vi "2048-1.vi"() -> ()   [LabVIEW 2018]
panel:
  out "Ring 25":u16(ring)
  out "Ring 24":u16(ring)
  out "Ring 23":u16(ring)
  out "Ring 22":u16(ring)
  out "Ring 21":u16(ring)
  out "Ring 20":u16(ring)
  out "Ring 19":u16(ring)
  out "Ring 18":u16(ring)
  out "Ring 17":u16(ring)
  out "Ring 16":u16(ring)
  out "Ring 15":u16(ring)
  out "Ring 14":u16(ring)
  out "Ring 13":u16(ring)
  out "Ring 12":u16(ring)
  out "Ring 11":u16(ring)
  out "Ring 10":u16(ring)
  out "Ring 9":u16(ring)
  out "Ring 8":u16(ring)
  out "Ring 7":u16(ring)
  out "Ring 6":u16(ring)
  out "Ring 5":u16(ring)
  out "Ring 4":u16(ring)
  out "Ring 3":u16(ring)
  out "Ring 2":u16(ring)
  out "mode":i32
  in  "Type":enum16{"經典", "角落動物", "星座", "寶可夢", "彩色"}(ring)
  out "ringArray":refnum<vi>[][](array[refnum])
  out "Ring":u16(ring)
  in  "Game Over":string="Game Over"
  in  "Winner":string="Winner"
  in  "New Game":bool
  out "Score":dbl
  in  "Exit":bool
  in  "Down":bool
  in  "Up":bool
  in  "Right":bool
  in  "Left":bool
  in  "Board":i32[][](array[numeric])=[[0, 0, 0, 0], [0, 0, 0, 0], [0, 0, 0, 0], [0, 0, 0, 0]]
  in  "Ring 26":u16(ring)
  # "Overview: This example is a LabVIEW version of the number game 2048.\nRequirements: LabVIEW 2012 (or compatible)\nInstructions:\n1.Run the VI\n2.Use the the left, right, up, and down arrows to slide number"
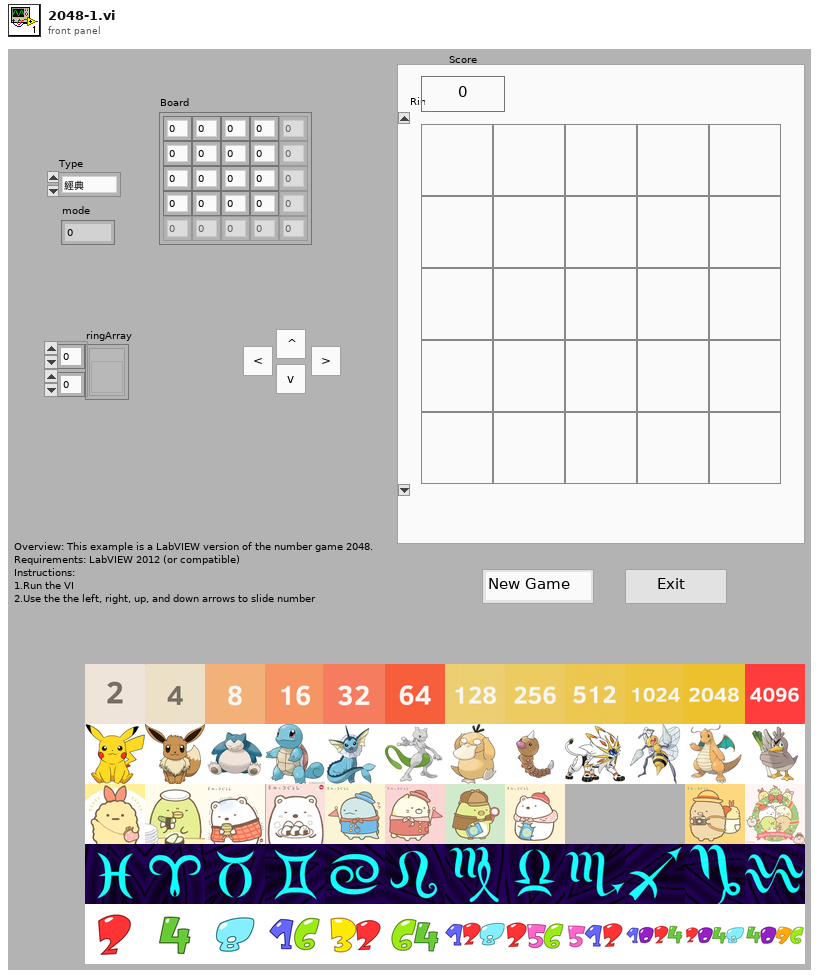
[diagram p1: front panel]
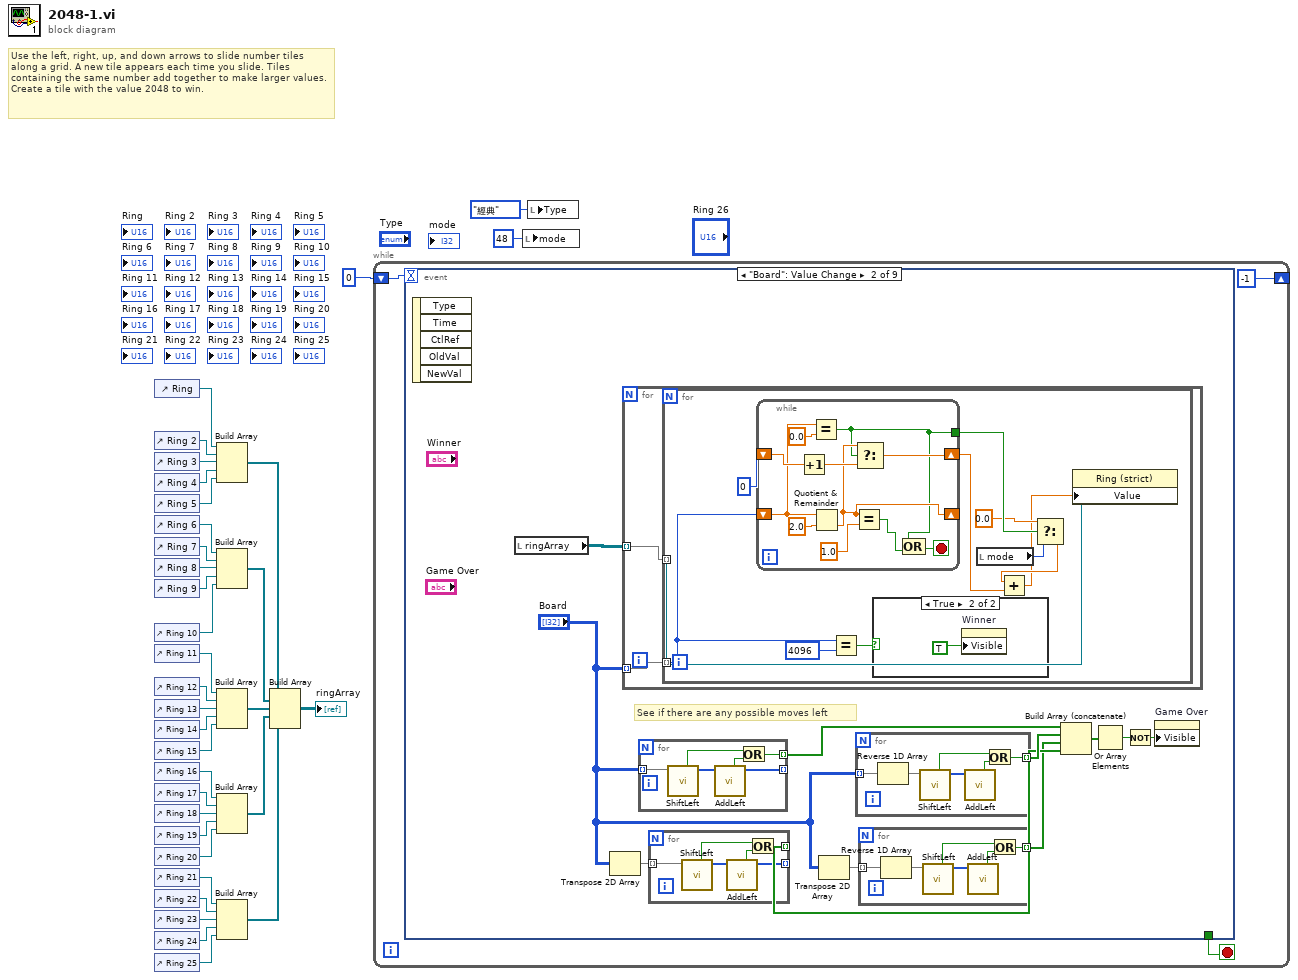
[diagram p0: block diagram]
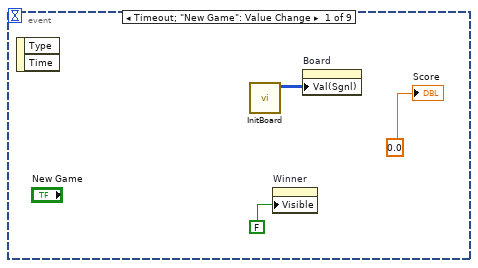
[diagram p2: hidden frame]
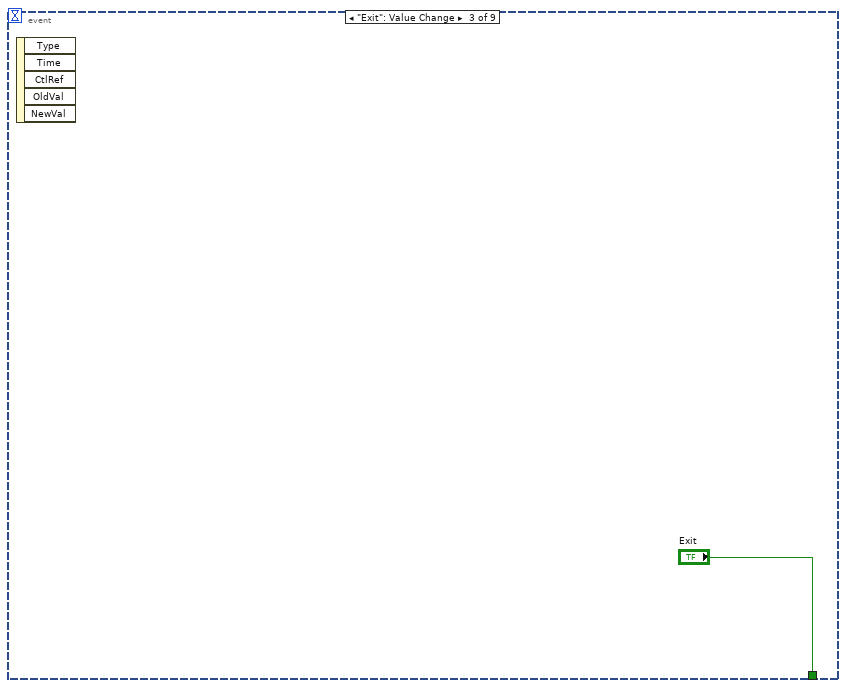
[diagram p4: hidden frame]
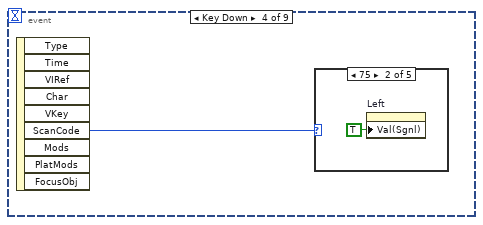
[diagram p5: hidden frame]
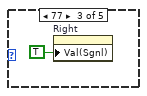
[diagram p7: hidden frame]
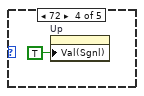
[diagram p8: hidden frame]
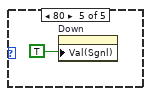
[diagram p9: hidden frame]
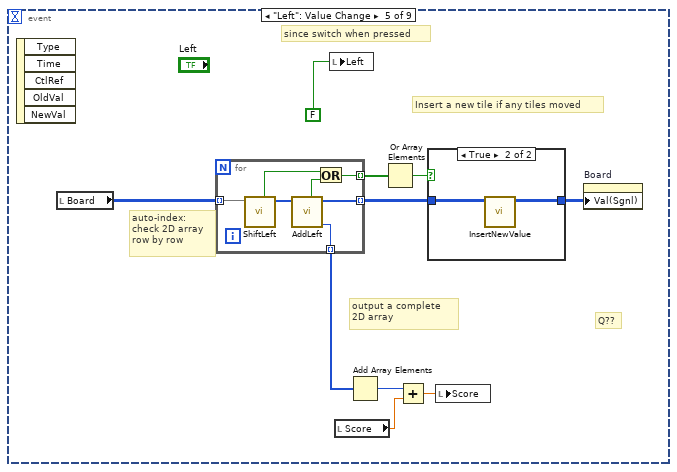
[diagram p10: hidden frame]
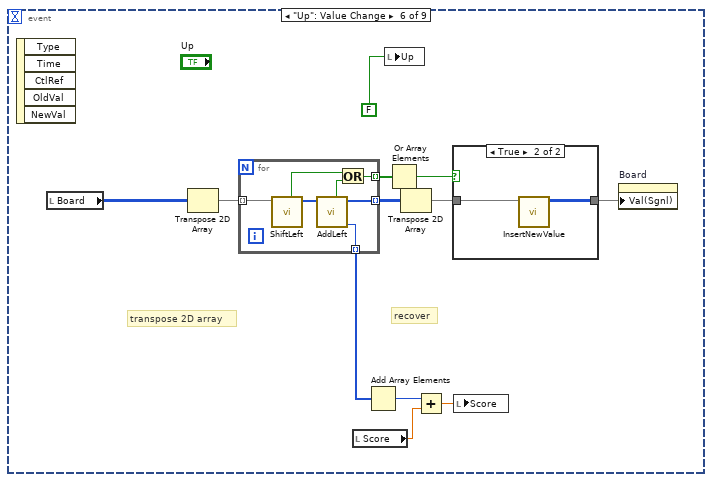
[diagram p12: hidden frame]
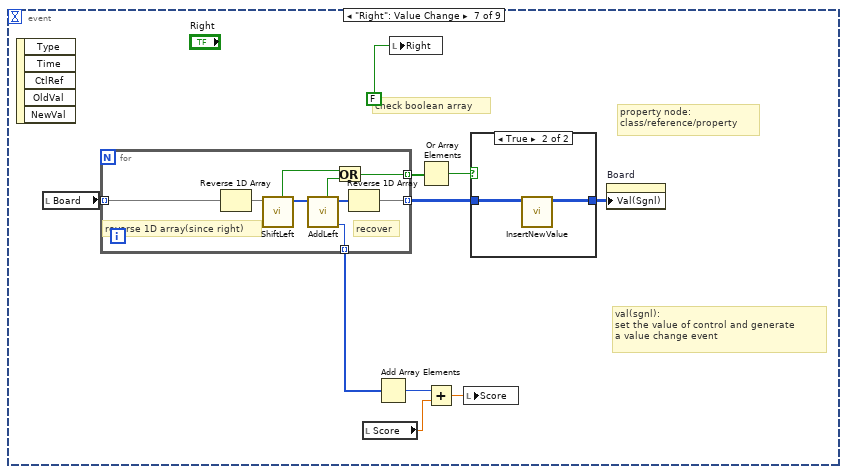
[diagram p14: hidden frame]
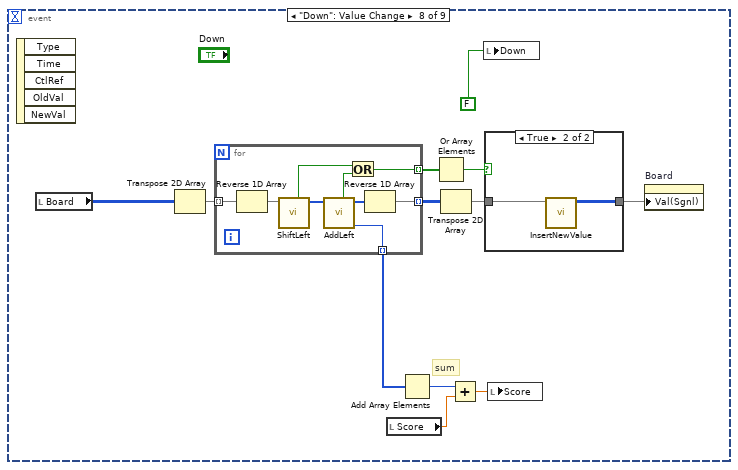
[diagram p16: hidden frame]
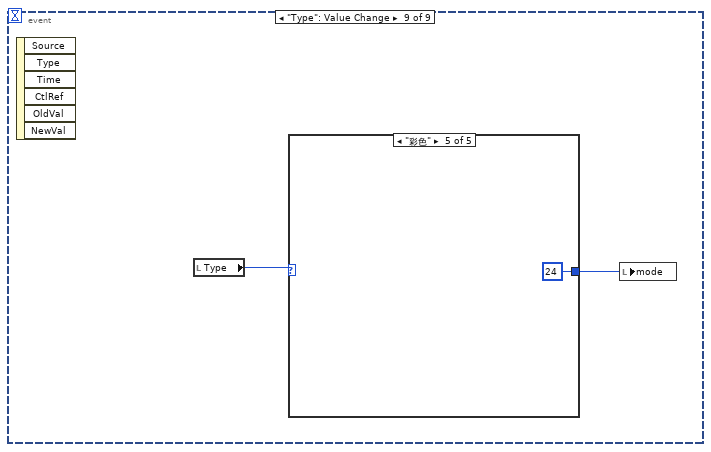
[diagram p18: hidden frame]
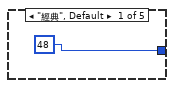
[diagram p19: hidden frame]
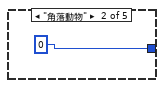
[diagram p20: hidden frame]
diagram:
  # "Use the left, right, up, and down arrows to slide number tiles along a grid. A new tile appears each time you slide. Tiles containing the same number add together to make larger values. Create a tile with the value 2048 to win."
  n1 = control-ref of="Ring"() -> (w32:refnum<vi>)
  n2 = control-ref of="Ring 2"() -> (w28:refnum<vi>)
  n3 = control-ref of="Ring 3"() -> (w29:refnum<vi>)
  n4 = control-ref of="Ring 4"() -> (w27:refnum<vi>)
  n5 = control-ref of="Ring 5"() -> (w26:refnum<vi>)
  n6 = control-ref of="Ring 6"() -> (w24:refnum<vi>)
  n7 = control-ref of="Ring 7"() -> (w23:refnum<vi>)
  n8 = control-ref of="Ring 8"() -> (w25:refnum<vi>)
  n9 = control-ref of="Ring 9"() -> (w22:refnum<vi>)
  n10 = control-ref of="Ring 10"() -> (w21:refnum<vi>)
  n11 = control-ref of="Ring 11"() -> (w20:refnum<vi>)
  n12 = control-ref of="Ring 12"() -> (w19:refnum<vi>)
  n13 = control-ref of="Ring 13"() -> (w18:refnum<vi>)
  n14 = control-ref of="Ring 14"() -> (w17:refnum<vi>)
  n15 = control-ref of="Ring 15"() -> (w16:refnum<vi>)
  n16 = control-ref of="Ring 16"() -> (w15:refnum<vi>)
  n17 = control-ref of="Ring 17"() -> (w14:refnum<vi>)
  n18 = control-ref of="Ring 18"() -> (w13:refnum<vi>)
  n19 = control-ref of="Ring 19"() -> (w12:refnum<vi>)
  n20 = control-ref of="Ring 20"() -> (w11:refnum<vi>)
  n21 = control-ref of="Ring 21"() -> (w10:refnum<vi>)
  n22 = control-ref of="Ring 22"() -> (w9:refnum<vi>)
  n23 = control-ref of="Ring 23"() -> (w8:refnum<vi>)
  n24 = control-ref of="Ring 24"() -> (w7:refnum<vi>)
  n25 = control-ref of="Ring 25"() -> (w6:refnum<vi>)
  n26 = Build Array(w32, w28, w29, w27, w26) -> (w33:refnum<vi>[])
  n27 = Build Array(w24, w23, w25, w22, w21) -> (w4:refnum<vi>[])
  n28 = Build Array(w20, w19, w18, w17, w16) -> (w5:refnum<vi>[])
  n29 = Build Array(w15, w14, w13, w12, w11) -> (w3:refnum<vi>[])
  n30 = Build Array(w10, w9, w8, w7, w6) -> (w2:refnum<vi>[])
  n31 = Build Array(w33, w4, w5, w3, w2) -> (→"ringArray":refnum<vi>[][])
  n32 = while {
    shift-right: [-1] -> _
    shift-left: 0 -> [w35]
    stop <- w37 stop-if-true
    n33 = event shown="[1] \"Board\": Value Change" {
      selector: _ -> [_ _ _ _ _ _ _ _ _]
      dyn-events: _ -> [_ _ _ _ _ _ _ _ _]
      timeout: w35 -> [_ _ _ _ _ _ _ _ _]
      tunnel: [_ _ "Exit" _ _ _ _ _ _] -> w37
      event Timeout; "New Game": Value Change {
        n34 = event-data() -> ()  [unwired: 1 in, 2 out]
        n35 = call "InitBoard.vi"() -> ("output array"=w39:i32[][])  [unwired: 11 in]
        n36 = property on="Winner" class="Str"("Visible"=FALSE) -> ()  [unwired: 2 in, 2 out]
        n37 = property on="Board" class="Arr (strict)"("Val(Sgnl)"=w39) -> ()  [unwired: 2 in, 2 out]
        "Score" <- 0.0 ("score")
      }
      event "Board": Value Change {
        # "See if there are any possible moves left"
        n38 = event-data() -> ()  [unwired: 1 in, 5 out]
        n39 = local read "ringArray"() -> (w41:refnum<vi>[][])
        n40 = Transpose 2D Array(2D array="Board") -> (transposed array=w51:i32[][])
        n41 = for {
          tunnel: "Board" -> [w76] mode=indexing
          tunnel: w41 -> [w77] mode=indexing
          n42 = for {
            tunnel: w77 -> [w88] mode=indexing
            tunnel: w76 -> [w80] mode=indexing
            n43 = while {
              shift-right: [w91] -> _
              shift-left: w80 -> [w96]
              shift-right: [w97] -> w85
              shift-left: 0 ("t") -> [w100]
              tunnel: [w90] -> w86
              stop <- w93 stop-if-true
              n44 = Increment(x=w100) -> (x+1=w98:dbl)
              n45 = Equal?(x=w96, y=0.0 ("f")) -> (x = y?=w90:bool)
              n46 = Quotient & Remainder(x=w96, y=2.0) -> (floor(x/y)=w91:dbl)  [unwired: 1 out]
              n47 = Equal?(x=w91, y=1.0) -> (x = y?=w94:bool)
              n48 = Select(t=w91, s=w90, f=w98) -> (s? t:f=w97:dbl)
              n49 = Compound Arithmetic op=OR(w90, w94) -> (w93:bool)
            }
            n50 = Equal?(x=w80, y=4096) -> (x = y?=w78:bool)
            n51 = case shown="True" w78 {
              frame False {
              }
              frame True {
                n52 = property on="Winner" class="Str"("Visible"=TRUE) -> ()  [unwired: 2 in, 2 out]
              }
            }
            n53 = local read "mode"() -> (w83:i32)
            n54 = Select(t=0.0, s=w86, f=w83) -> (s? t:f=w82:dbl)
            n55 = Add(x=w82, y=w85) -> (x+y=w81:dbl)
            n56 = property class="Ring (strict)"(reference=w88, "Value"=w81) -> ()  [unwired: 1 in, 2 out]
          }
        }
        n57 = for {
          tunnel: "Board" -> [w75] mode=indexing
          tunnel: [w73] -> _ mode=indexing
          tunnel: [w70] -> w48 mode=indexing
          n58 = call "ShiftLeft.vi"("Array"=w75) -> ("Array 2"=w74:i32[], "tiles moved?"=w71:bool)  [unwired: 9 in]
          n59 = call "AddLeft.vi"("Array"=w74) -> ("Array 2"=w73:i32[], "tiles moved?"=w72:bool)  [unwired: 8 in, 1 out]
          n60 = Or(x=w71, y=w72) -> (x .or. y?=w70:bool)
        }
        n61 = for {
          tunnel: w51 -> [w69] mode=indexing
          tunnel: [w67] -> _ mode=indexing
          tunnel: [w64] -> w46 mode=indexing
          n62 = call "ShiftLeft.vi"("Array"=w69) -> ("Array 2"=w68:i32[], "tiles moved?"=w65:bool)  [unwired: 9 in]
          n63 = call "AddLeft.vi"("Array"=w68) -> ("Array 2"=w67:i32[], "tiles moved?"=w66:bool)  [unwired: 8 in, 1 out]
          n64 = Or(x=w65, y=w66) -> (x .or. y?=w64:bool)
        }
        n65 = Transpose 2D Array(2D array="Board") -> (transposed array=w50:i32[][])
        n66 = for {
          tunnel: "Board" -> [w62] mode=indexing
          tunnel: [w58] -> w47 mode=indexing
          n67 = Reverse 1D Array(array=w62) -> (reversed array=w61:i32[])
          n68 = call "ShiftLeft.vi"("Array"=w61) -> ("Array 2"=w63:i32[], "tiles moved?"=w59:bool)  [unwired: 9 in]
          n69 = call "AddLeft.vi"("Array"=w63) -> ("tiles moved?"=w60:bool)  [unwired: 8 in, 2 out]
          n70 = Or(x=w59, y=w60) -> (x .or. y?=w58:bool)
        }
        n71 = for {
          tunnel: w50 -> [w56] mode=indexing
          tunnel: [w52] -> w45 mode=indexing
          n72 = Reverse 1D Array(array=w56) -> (reversed array=w55:i32[])
          n73 = call "ShiftLeft.vi"("Array"=w55) -> ("Array 2"=w57:i32[], "tiles moved?"=w53:bool)  [unwired: 9 in]
          n74 = call "AddLeft.vi"("Array"=w57) -> ("tiles moved?"=w54:bool)  [unwired: 8 in, 2 out]
          n75 = Or(x=w53, y=w54) -> (x .or. y?=w52:bool)
        }
        n76 = Build Array (concatenate)(w48, w47, w45, w46) -> (w44:bool[])
        n77 = Or Array Elements(Boolean array=w44) -> (logical OR=w43:bool)
        n78 = Not(x=w43) -> (.not. x?=w42:bool)
        n79 = property on="Game Over" class="Str"("Visible"=w42) -> ()  [unwired: 2 in, 2 out]
      }
      event "Exit": Value Change {
        n80 = event-data() -> ()  [unwired: 1 in, 5 out]
      }
      event Key Down {
        n81 = event-data() -> ("ScanCode"=w102:i16)  [unwired: 1 in, 8 out]
        n82 = case shown="75" w102 {
          frame 0, Default {
          }
          frame 75 {
            n83 = property on="Left" class="Bool (strict)"("Val(Sgnl)"=TRUE) -> ()  [unwired: 2 in, 2 out]
          }
          frame 77 {
            n84 = property on="Right" class="Bool (strict)"("Val(Sgnl)"=TRUE) -> ()  [unwired: 2 in, 2 out]
          }
          frame 72 {
            n85 = property on="Up" class="Bool (strict)"("Val(Sgnl)"=TRUE) -> ()  [unwired: 2 in, 2 out]
          }
          frame 80 {
            n86 = property on="Down" class="Bool (strict)"("Val(Sgnl)"=TRUE) -> ()  [unwired: 2 in, 2 out]
          }
        }
      }
      event "Left": Value Change {
        # "output a complete\n2D array"
        # "auto-index:\ncheck 2D array\nrow by row"
        # "since switch when pressed"
        # "Q??"
        # "Insert a new tile if any tiles moved"
        n87 = event-data() -> ()  [unwired: 1 in, 5 out]
        n88 = local read "Board"() -> (w115:i32[][])
        n89 = for {
          tunnel: w115 -> [w126] mode=indexing
          tunnel: [w124] -> w114 mode=indexing
          tunnel: [w123] -> w110 mode=indexing
          tunnel: [w120] -> w108 mode=indexing
          n90 = call "ShiftLeft.vi"("Array"=w126) -> ("Array 2"=w125:i32[], "tiles moved?"=w121:bool)  [unwired: 9 in]
          n91 = call "AddLeft.vi"("Array"=w125) -> ("score"=w123:i32, "Array 2"=w124:i32[], "tiles moved?"=w122:bool)  [unwired: 8 in]
          n92 = Or(x=w121, y=w122) -> (x .or. y?=w120:bool)
        }
        n93 = local write "Left"(FALSE ("Left")) -> ()
        n94 = local read "Score"() -> (w111:dbl)
        n95 = Add Array Elements(numeric array=w110) -> (sum=w113:i32)
        n96 = Or Array Elements(Boolean array=w108) -> (logical OR=w107:bool)
        n97 = Add(x=w113, y=w111) -> (x+y=w112:dbl)
        n98 = case shown="True" w107 {
          tunnel: w114 -> [w117 w119]
          tunnel: [w117 w118] -> w109
          frame False {
          }
          frame True {
            n99 = call "InsertNewValue.vi"("Board"=w119) -> ("output"=w118:i32[][])  [unwired: 10 in]
          }
        }
        n100 = local write "Score"(w112) -> ()
        n101 = property on="Board" class="Arr (strict)"("Val(Sgnl)"=w109) -> ()  [unwired: 2 in, 2 out]
      }
      event "Up": Value Change {
        # "recover"
        # "transpose 2D array"
        n102 = event-data() -> ()  [unwired: 1 in, 5 out]
        n103 = local read "Board"() -> (w137:i32[][])
        n104 = Transpose 2D Array(2D array=w137) -> (transposed array=w135:i32[][])
        n105 = for {
          tunnel: w135 -> [w148] mode=indexing
          tunnel: [w146] -> w136 mode=indexing
          tunnel: [w145] -> w130 mode=indexing
          tunnel: [w142] -> w128 mode=indexing
          n106 = call "ShiftLeft.vi"("Array"=w148) -> ("Array 2"=w147:i32[], "tiles moved?"=w143:bool)  [unwired: 9 in]
          n107 = call "AddLeft.vi"("Array"=w147) -> ("score"=w145:i32, "Array 2"=w146:i32[], "tiles moved?"=w144:bool)  [unwired: 8 in]
          n108 = Or(x=w143, y=w144) -> (x .or. y?=w142:bool)
        }
        n109 = local read "Score"() -> (w131:dbl)
        n110 = Add Array Elements(numeric array=w130) -> (sum=w133:i32)
        n111 = local write "Up"(FALSE ("Up")) -> ()
        n112 = Or Array Elements(Boolean array=w128) -> (logical OR=w127:bool)
        n113 = Transpose 2D Array(2D array=w136) -> (transposed array=w134:i32[][])
        n114 = Add(x=w133, y=w131) -> (x+y=w132:dbl)
        n115 = case shown="True" w127 {
          tunnel: w134 -> [w139 w141]
          tunnel: [w139 w140] -> w129
          frame False {
          }
          frame True {
            n116 = call "InsertNewValue.vi"("Board"=w141) -> ("output"=w140:i32[][])  [unwired: 10 in]
          }
        }
        n117 = local write "Score"(w132) -> ()
        n118 = property on="Board" class="Arr (strict)"("Val(Sgnl)"=w129) -> ()  [unwired: 2 in, 2 out]
      }
      event "Right": Value Change {
        # "check boolean array"
        # "property node:\nclass/reference/property"
        # "val(sgnl):\nset the value of control and generate \na value change event"
        n119 = event-data() -> ()  [unwired: 1 in, 5 out]
        n120 = local read "Board"() -> (w157:i32[][])
        n121 = for {
          tunnel: w157 -> [w168] mode=indexing
          tunnel: [w166] -> w156 mode=indexing
          tunnel: [w165] -> w152 mode=indexing
          tunnel: [w162] -> w150 mode=indexing
          # "reverse 1D array(since right)"
          # "recover"
          n122 = Reverse 1D Array(array=w168) -> (reversed array=w167:i32[])
          n123 = call "ShiftLeft.vi"("Array"=w167) -> ("Array 2"=w170:i32[], "tiles moved?"=w163:bool)  [unwired: 9 in]
          n124 = call "AddLeft.vi"("Array"=w170) -> ("score"=w165:i32, "Array 2"=w169:i32[], "tiles moved?"=w164:bool)  [unwired: 8 in]
          n125 = Or(x=w163, y=w164) -> (x .or. y?=w162:bool)
          n126 = Reverse 1D Array(array=w169) -> (reversed array=w166:i32[])
        }
        n127 = local read "Score"() -> (w153:dbl)
        n128 = Add Array Elements(numeric array=w152) -> (sum=w155:i32)
        n129 = local write "Right"(FALSE ("Right")) -> ()
        n130 = Or Array Elements(Boolean array=w150) -> (logical OR=w149:bool)
        n131 = Add(x=w155, y=w153) -> (x+y=w154:dbl)
        n132 = local write "Score"(w154) -> ()
        n133 = case shown="True" w149 {
          tunnel: w156 -> [w159 w161]
          tunnel: [w159 w160] -> w151
          frame False {
          }
          frame True {
            n134 = call "InsertNewValue.vi"("Board"=w161) -> ("output"=w160:i32[][])  [unwired: 10 in]
          }
        }
        n135 = property on="Board" class="Arr (strict)"("Val(Sgnl)"=w151) -> ()  [unwired: 2 in, 2 out]
      }
      event "Down": Value Change {
        # "sum"
        n136 = event-data() -> ()  [unwired: 1 in, 5 out]
        n137 = local read "Board"() -> (w181:i32[][])
        n138 = Transpose 2D Array(2D array=w181) -> (transposed array=w179:i32[][])
        n139 = for {
          tunnel: w179 -> [w192] mode=indexing
          tunnel: [w190] -> w180 mode=indexing
          tunnel: [w189] -> w177 mode=indexing
          tunnel: [w186] -> w172 mode=indexing
          n140 = Reverse 1D Array(array=w192) -> (reversed array=w191:i32[])
          n141 = call "ShiftLeft.vi"("Array"=w191) -> ("Array 2"=w194:i32[], "tiles moved?"=w187:bool)  [unwired: 9 in]
          n142 = call "AddLeft.vi"("Array"=w194) -> ("score"=w189:i32, "Array 2"=w193:i32[], "tiles moved?"=w188:bool)  [unwired: 8 in]
          n143 = Or(x=w187, y=w188) -> (x .or. y?=w186:bool)
          n144 = Reverse 1D Array(array=w193) -> (reversed array=w190:i32[])
        }
        n145 = local read "Score"() -> (w174:dbl)
        n146 = Add Array Elements(numeric array=w177) -> (sum=w176:i32)
        n147 = Or Array Elements(Boolean array=w172) -> (logical OR=w171:bool)
        n148 = Transpose 2D Array(2D array=w180) -> (transposed array=w178:i32[][])
        n149 = Add(x=w176, y=w174) -> (x+y=w175:dbl)
        n150 = local write "Down"(FALSE ("Down")) -> ()
        n151 = case shown="True" w171 {
          tunnel: w178 -> [w183 w185]
          tunnel: [w183 w184] -> w173
          frame False {
          }
          frame True {
            n152 = call "InsertNewValue.vi"("Board"=w185) -> ("output"=w184:i32[][])  [unwired: 10 in]
          }
        }
        n153 = local write "Score"(w175) -> ()
        n154 = property on="Board" class="Arr (strict)"("Val(Sgnl)"=w173) -> ()  [unwired: 2 in, 2 out]
      }
      event "Type": Value Change {
        n155 = event-data() -> ()  [unwired: 1 in, 6 out]
        n156 = local read "Type"() -> (w196:enum16{"經典", "角落動物", "星座", "寶可夢", "彩色"})
        n157 = case shown="\"彩色\"" w196 {
          tunnel: [48 0 12 36 24] -> w195
          frame "經典", Default {
          }
          frame "角落動物" {
          }
          frame "星座" {
          }
          frame "寶可夢" {
          }
          frame "彩色" {
          }
        }
        n158 = local write "mode"(w195) -> ()
      }
    }
  }
  n159 = local write "mode"(48 ("mode")) -> ()
  n160 = local write "Type"(enum16{"經典", "角落動物", "星座", "寶可夢", "彩色"}."經典" ("Type")) -> ()
